vi "LJM logger config panel load and read register list.vi"(6 "Streaming App?":bool=TRUE, 9 "App name":string="LJM_New_Open", 10 "Working Directory":path, 11 "Handle In":i32) -> (0 "Error Out":errorcluster, 1 "Register Values":dbl[](array[numeric]) format="%.2f", 2 "Register List":string[](array[string]), 3 "Handle Out":i32, 5 "Register List Config Filename":string)   [LabVIEW 2026]
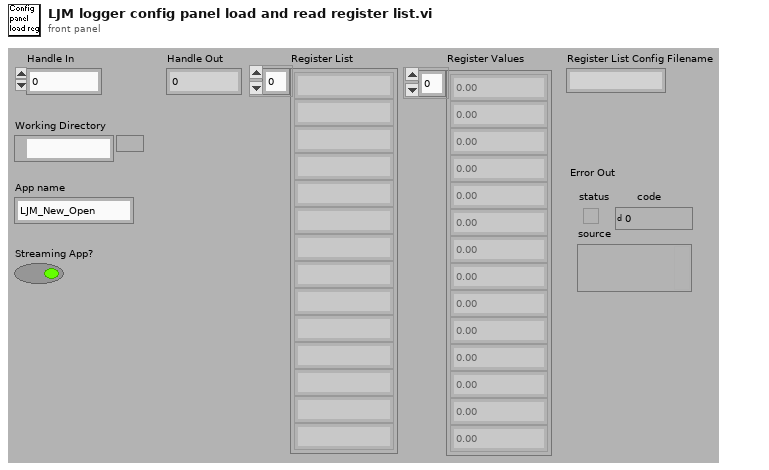
[diagram p1: front panel]
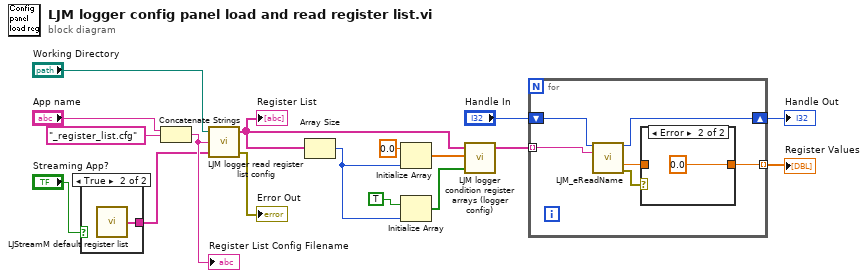
[diagram p0: block diagram]
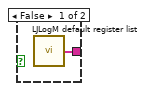
[diagram p2: hidden frame]
diagram:
  n1 = case shown="True" "Streaming App?" {
    tunnel: [w18 w19] -> w2
    frame False {
      n2 = call "LJLogM default register list.vi"() -> ("Default Register List"=w18:string[])  [unwired: 1 in]
    }
    frame True {
      n3 = call "LJStreamM default register list.vi"() -> ("Default Register List"=w19:string[])  [unwired: 1 in]
    }
  }
  n4 = Concatenate Strings("App name", "_register_list.cfg" ("string")) -> (w15:string)
  "Register List Config Filename" <- w15
  n5 = call "LJM logger read register list config.vi"("Default Register List"=w2, "filename"=w15, "Working Directory"="Working Directory") -> ("error out"=→"Error Out":errorcluster, "Register List"=w14:string[])  [unwired: 1 out]
  "Register List" <- w14
  n6 = Array Size(array=w14) -> (size(s)=w10:i32)
  n7 = Initialize Array(0.0, w10) -> (w11:dbl[])
  n8 = Initialize Array(TRUE, w10) -> (w12:bool[])
  n9 = call "LJM logger condition register arrays (logger config).vi"("Access?"=w12, "Values"=w11, "Names"=w14) -> ("Names Out"=w8:string[])  [unwired: 1 in, 1 out]
  n10 = for {
    tunnel: w8 -> [w24] mode=indexing
    shift-right: [w21] -> w6
    shift-left: "Handle In" -> [w25]
    tunnel: [w20] -> w5 mode=indexing
    n11 = call "LJM_eReadName.vi"("Handle In"=w25, "Name"=w24) -> ("Handle Out"=w21:i32, "Value"=w22:dbl, "error out"=w23:errorcluster)  [unwired: 11 in]
    n12 = case shown="Error" w23 {
      tunnel: w22 -> [w26 _]
      tunnel: [w26 0.0 ("Value")] -> w20
      frame No Error {
      }
      frame Error {
      }
    }
  }
  "Handle Out" <- w6
  "Register Values" <- w5
